vi "PicoScopeospaUnitInfo.vi"(8 "error in (no error)":errorcluster, 11 "handle in":i16) -> (0 "error out":errorcluster, 2 "Unit Info":T1, 3 "handle out":i16)   [LabVIEW 2009]
doc: "Returns Driver and Unit Information"
uses:
  psospa.dll
panel:
  out "json string":string
  out "outputStringLength":i32
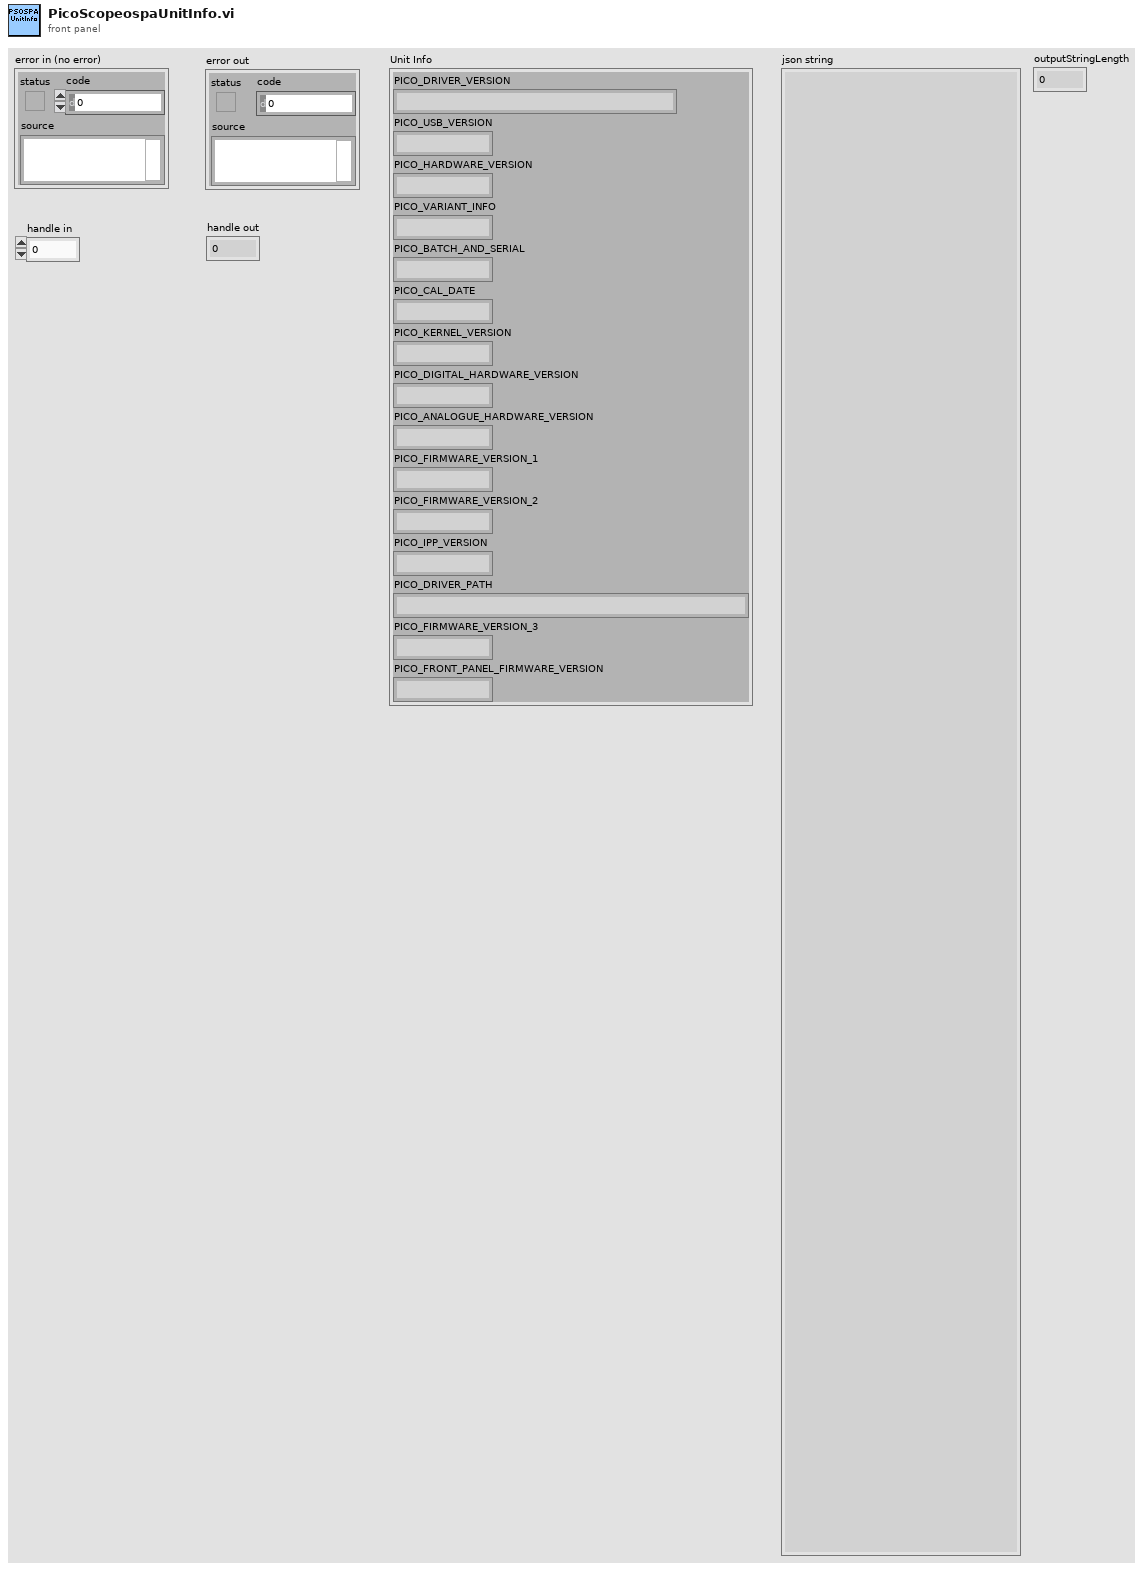
[diagram p1: front panel]
types:
  T1 = cluster{"PICO_DRIVER_VERSION":string, "PICO_USB_VERSION":string, "PICO_HARDWARE_VERSION":string, "PICO_VARIANT_INFO":string, "PICO_BATCH_AND_SERIAL":string, "PICO_CAL_DATE":string, "PICO_KERNEL_VERSION":string, "PICO_DIGITAL_HARDWARE_VERSION":string, "PICO_ANALOGUE_HARDWARE_VERSION":string, "PICO_FIRMWARE_VERSION_1":string, "PICO_FIRMWARE_VERSION_2":string, "PICO_IPP_VERSION":string, "PICO_DRIVER_PATH":string, "PICO_FIRMWARE_VERSION_3":string, "PICO_FRONT_PANEL_FIRMWARE_VERSION":string}
  T2 = cluster{"[0]":string, "[1]":string, "[2]":string, "[3]":string, "[4]":string, "[5]":string, "[6]":string, "[7]":string, "[8]":string, "[9]":string, "[10]":string, "[11]":string, "[12]":string, "[13]":string, "[14]":string}
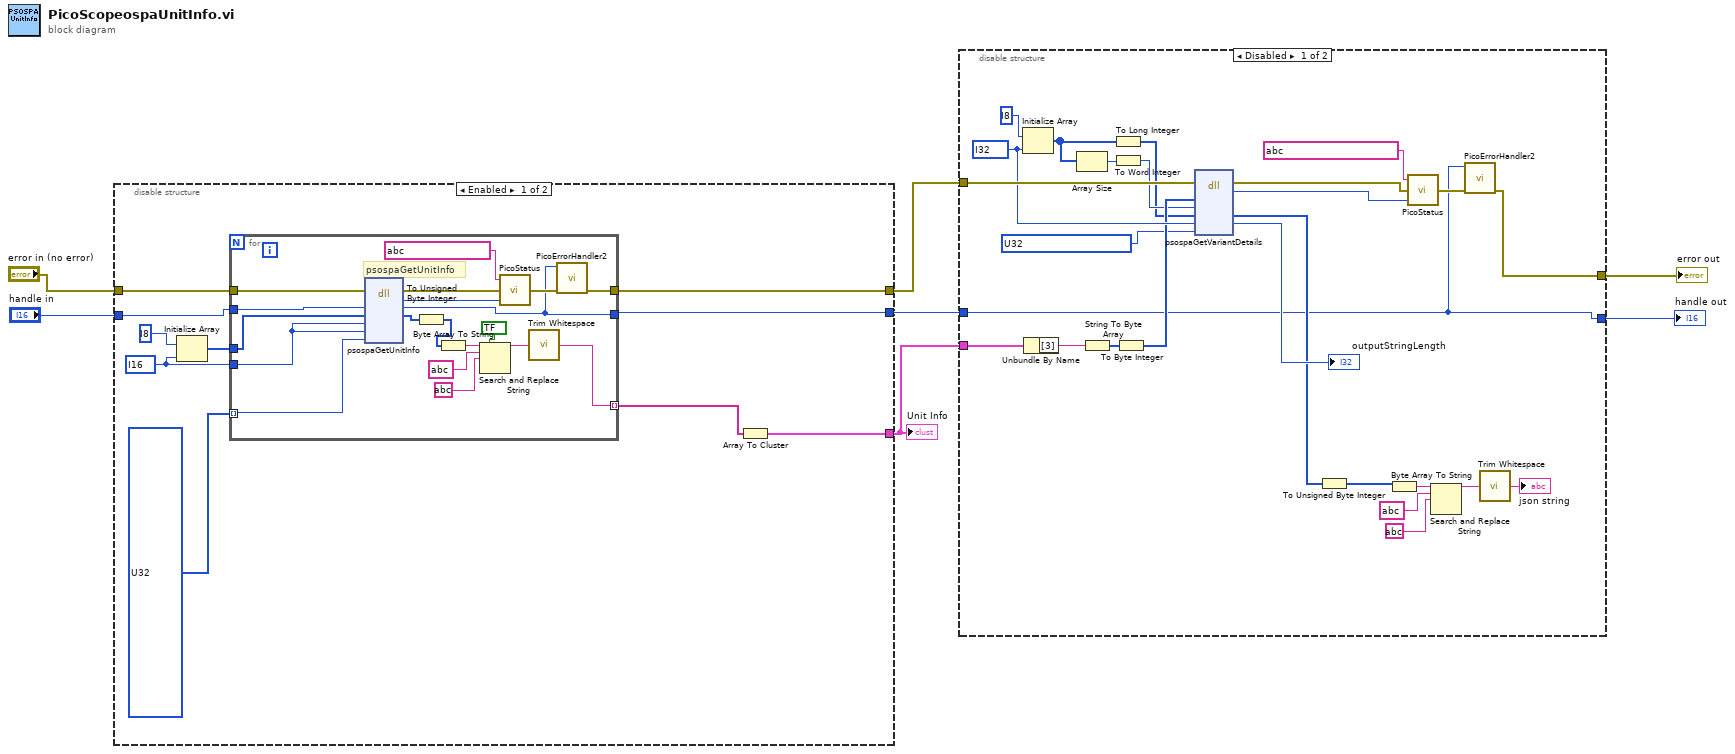
[diagram p0: block diagram]
diagram:
  n1 = disable-structure shown="Enabled" {
    disable-tunnel: "error in (no error)" -> [w14 w38]
    disable-tunnel: "handle in" -> [w13 w37]
    disable-tunnel: [w12 w37] -> w2
    disable-tunnel: [w11 w38] -> w4
    disable-tunnel: [w8 _] -> w3
    frame #0 {
      w15 = i16 ? ("requiredSize")
      n2 = Initialize Array(i8 ? ("element"), w15) -> (w17:i8[])
      n3 = for {
        tunnel: w14 -> [w30]
        tunnel: [w19] -> w11
        tunnel: w17 -> [w31]
        tunnel: w13 -> [w29]
        tunnel: w15 -> [w28]
        tunnel: [w22] -> w12
        tunnel: u32[] ? ("initialized array") -> [w24] mode=indexing
        tunnel: [w21] -> w10 mode=indexing
        # "psospaGetUnitInfo"
        n4 = dll-call lib="psospa.dll" fn="psospaGetUnitInfo"(error in=w30, "handle"=w29, "string"=w31, "stringLength"=w28, "requiredSize"=w28, "deviceInfo"=w24) -> (error out=w20:errorcluster, "PICO_STATUS"=w18:u32, "handle"=w22:i16, "string"=w26:i8[])  [unwired: 5 in, 1 out]
        n5 = To Unsigned Byte Integer(number=w26) -> (unsigned 8bit integer=w25:u8[])
        n6 = Byte Array To String(unsigned byte array=w25) -> (string=w35:string)
        n7 = Search and Replace String(replace all?=bool ? ("replace all? (F)"), input string=w35, search string=string ?, replace string=string ?) -> (result string=w34:string)  [unwired: 4 in, 3 out]
        n8 = call "PicoStatus.vi"("PICO STATUS"=w18, "error in"=w20, "source"=string ?) -> ("error out"=w23:errorcluster)
        n9 = call <vilib>:"Trim Whitespace.vi"("string"=w34) -> ("trimmed string"=w21:string)  [unwired: 1 in]
        n10 = call "PicoErrorHandler2.vi"("error in (no error)"=w23, "handle In"=w22) -> ("error out"=w19:errorcluster)  [unwired: 9 in]
      }
      n11 = Array To Cluster(array=w10) -> (cluster=w8:T2)
    }
    frame #1 {
    }
  }
  "Unit Info" <- w3
  n12 = disable-structure shown="Disabled" {
    disable-tunnel: [w60 w65] -> w5
    disable-tunnel: w4 -> [w59 w65]
    disable-tunnel: w3 -> [w56 _]
    disable-tunnel: w2 -> [w39 w66]
    disable-tunnel: [w39 w66] -> w1
    frame #0 {
      w40 = u32 ? items=["PICO_JSON_DATA", "PICO_JSON_SCHEMA"] ("PICO_TEXT_FORMAT")
      w57 = i32 ? ("dimension size")
      n13 = Initialize Array(i8 ? ("element"), w57) -> (w42:i8[])
      n14 = Unbundle By Name(w56) -> ("[3]"=w55:string)
      n15 = Array Size(array=w42) -> (size(s)=w43:i32)
      n16 = String To Byte Array(string=w55) -> (unsigned byte array=w54:u8[])
      n17 = To Long Integer(number=w42) -> (32bit integer=w41:i32[])
      n18 = To Word Integer(number=w43) -> (16bit integer=w44:i16)
      n19 = To Byte Integer(number=w54) -> (8bit integer=w53:i8[])
      n20 = dll-call lib="psospa.dll" fn="psospaGetVariantDetails"(error in=w59, "variantName"=w53, "variantNameLength"=w44, "outputString"=w41, "outputStringLength"=w57, "textFormat"=w40) -> (error out=w62:errorcluster, "PICO_STATUS"=w61:u32, "outputString"=w46:i32[], "outputStringLength"=→"outputStringLength":i32)  [unwired: 5 in, 1 out]
      n21 = To Unsigned Byte Integer(number=w46) -> (unsigned 8bit integer=w47:u8[])
      n22 = Byte Array To String(unsigned byte array=w47) -> (string=w50:string)
      n23 = call "PicoStatus.vi"("PICO STATUS"=w61, "error in"=w62, "source"=string ?) -> ("error out"=w63:errorcluster)
      n24 = Search and Replace String(input string=w50, search string=string ?, replace string=string ?) -> (result string=w49:string)  [unwired: 5 in, 3 out]
      n25 = call "PicoErrorHandler2.vi"("error in (no error)"=w63, "handle In"=w39) -> ("error out"=w60:errorcluster)  [unwired: 9 in]
      n26 = call <vilib>:"Trim Whitespace.vi"("string"=w49) -> ("trimmed string"=→"json string":string)  [unwired: 1 in]
    }
    frame #1 {
    }
  }
  "error out" <- w5
  "handle out" <- w1
